vi "calc_velocity.vi"(9 "Time per cell":dbl, 10 "Path length":dbl, 11 "Neurons":u16) -> (3 "Velocity":dbl)   [LabVIEW 2010]
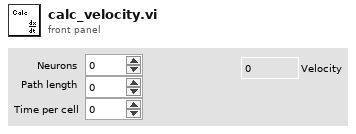
[diagram p1: front panel]
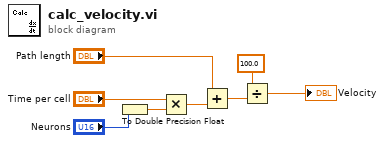
[diagram p0: block diagram]
diagram:
  n1 = To Double Precision Float(number="Neurons") -> (double precision float=w5:dbl)
  n2 = Multiply(x="Time per cell", y=w5) -> (x*y=w2:dbl)
  n3 = Add(x="Path length", y=w2) -> (x+y=w6:dbl)
  n4 = Divide(x=100.0, y=w6) -> (x/y=→"Velocity":dbl)
